vi "OPEN.vi"(10 "Input Data":dbl[](array[numeric]), 11 "Mean In":dbl=1600.0) -> (3 "OPEN":bool)   [LabVIEW 2012]
panel:
  out "Diff":dbl
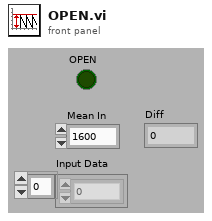
[diagram p1: front panel]
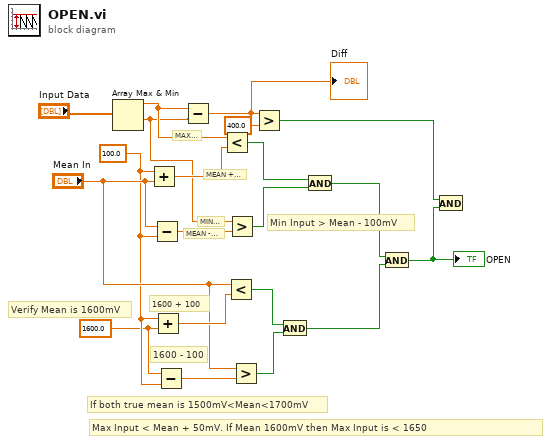
[diagram p0: block diagram]
diagram:
  w13 = 1600.0
  w14 = 100.0
  # "1600 + 100"
  # "1600 - 100"
  # "MEAN + 100"
  # "MAXVAL"
  # "MINVAL"
  # "MEAN - 100"
  # "Min Input > Mean - 100mV"
  # "Max Input < Mean + 50mV. If Mean 1600mV then Max Input is < 1650"
  # "If both true mean is 1500mV<Mean<1700mV"
  # "Verify Mean is 1600mV"
  n1 = Array Max & Min(array="Input Data") -> (max value=w6:dbl, min value=w5:dbl)  [unwired: 2 out]
  n2 = Add(x=w14, y="Mean In") -> (x+y=w20:dbl)
  n3 = Subtract(x="Mean In", y=w14) -> (x-y=w19:dbl)
  n4 = Add(x=w14, y=w13) -> (x+y=w17:dbl)
  n5 = Subtract(x=w13, y=w14) -> (x-y=w16:dbl)
  n6 = Subtract(x=w6, y=w5) -> (x-y=w2:dbl)
  "Diff" <- w2
  n7 = Less?(x=w6, y=w20) -> (x < y?=w12:bool)
  n8 = Less?(x="Mean In", y=w17) -> (x < y?=w10:bool)
  n9 = Greater?(x=w5, y=w19) -> (0:w11:bool)
  n10 = Greater?(x="Mean In", y=w16) -> (0:w9:bool)
  n11 = Greater?(x=w2, y=400.0) -> (0:w3:bool)
  n12 = And(x=w10, y=w9) -> (x .and. y?=w7:bool)
  n13 = And(x=w12, y=w11) -> (x .and. y?=w8:bool)
  n14 = And(x=w8, y=w7) -> (x .and. y?=w1:bool)
  "OPEN" <- w1
  n15 = And(x=w3, y=w1) -> ()  [unwired: 1 out]
